vi "Little Digit Main.vi"() -> ()   [LabVIEW 2018]
uses:
  <vilib>/Instr/_visa.llb/VISA Configure Serial Port (Instr).vi
  <vilib>/Utility/inputDevices.llb/joystickAcquire.vi
  <vilib>/Utility/inputDevices.llb/closeJoystick.vi
  <vilib>/ptbypt/NI_PtbyPt.lvlib
panel:
  out "Elbow Degrees":dbl format="%.2f"
  out "Shoulder Degrees":dbl format="%.2f"
  in  "Vector Mode":bool=TRUE
  out "Shoulder Power":dbl
  out "Y axis":i32
  out "Z axis":i32
  out "Elbow power":dbl
  out "joystick info":T1(array[cluster])=[{"axes total"=6, "buttons total"=2, "pov total"=0, "device name"="SpaceNavigator"}, {"axes total"=8, "buttons total"=128, "pov total"=0, "device name"="Tetherscript Virtual Controller"}, {"axes total"=7, "buttons total"=4, "pov total"=1, "device name"="3Dconnexion KMJ Emulator"}]
  in  "OK Button":bool
  out "Lap Times":dbl[](array[numeric])
  out "Elapsed Time (s)":dbl=6.446096897125244
  out "Rotation Counts":i32=123
  out "Shoulder Counts":i32=65
  out "Elbow Counts":i32=112
  out "Wrist Counts":i32=80
  out "axis info":T2={"X axis"=-2, "Y axis"=-2, "Z axis"=-2, "X axis rotation"=-2, "Y axis rotation"=-2, "Z axis rotation"=-2, "U axis"=-2, "V axis"=-2}
  in  "stop":bool
  # "Little Digit\nTeam 5013"
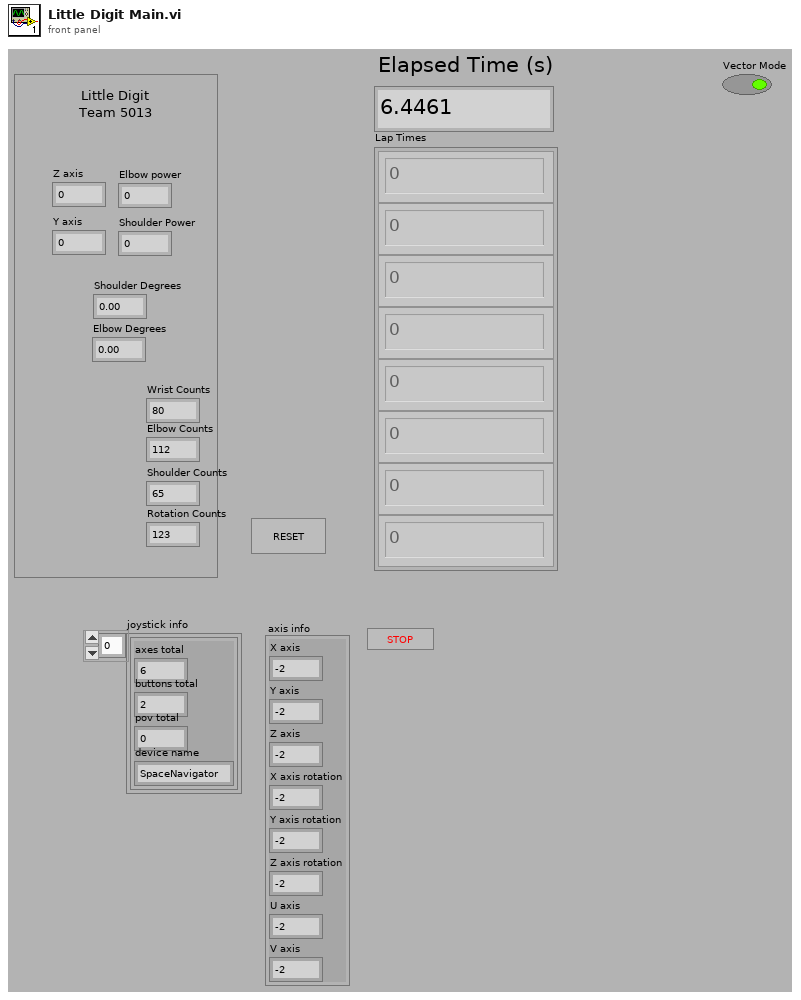
[diagram p1: front panel]
types:
  T1 = cluster{"axes total":u32, "buttons total":u32, "pov total":u32, "device name":string}[]
  T2 = cluster{"X axis":i32, "Y axis":i32, "Z axis":i32, "X axis rotation":i32, "Y axis rotation":i32, "Z axis rotation":i32, "U axis":i32, "V axis":i32}
  T3 = cluster{"button 1":bool, "button 2":bool, "button 3":bool, "button 4":bool, "button 5":bool, "button 6":bool, "button 7":bool, "button 8":bool, "button 9":bool, "button 10":bool, "button 11":bool, "button 12":bool, "button 13":bool, "button 14":bool, "button 15":bool, "button 16":bool, "button 17":bool, "button 18":bool, "button 19":bool, "button 20":bool, "button 21":bool, "button 22":bool, "button 23":bool, "button 24":bool, "button 25":bool, "button 26":bool, "button 27":bool, "button 28":bool, "button 29":bool, "button 30":bool, "button 31":bool, "button 32":bool}
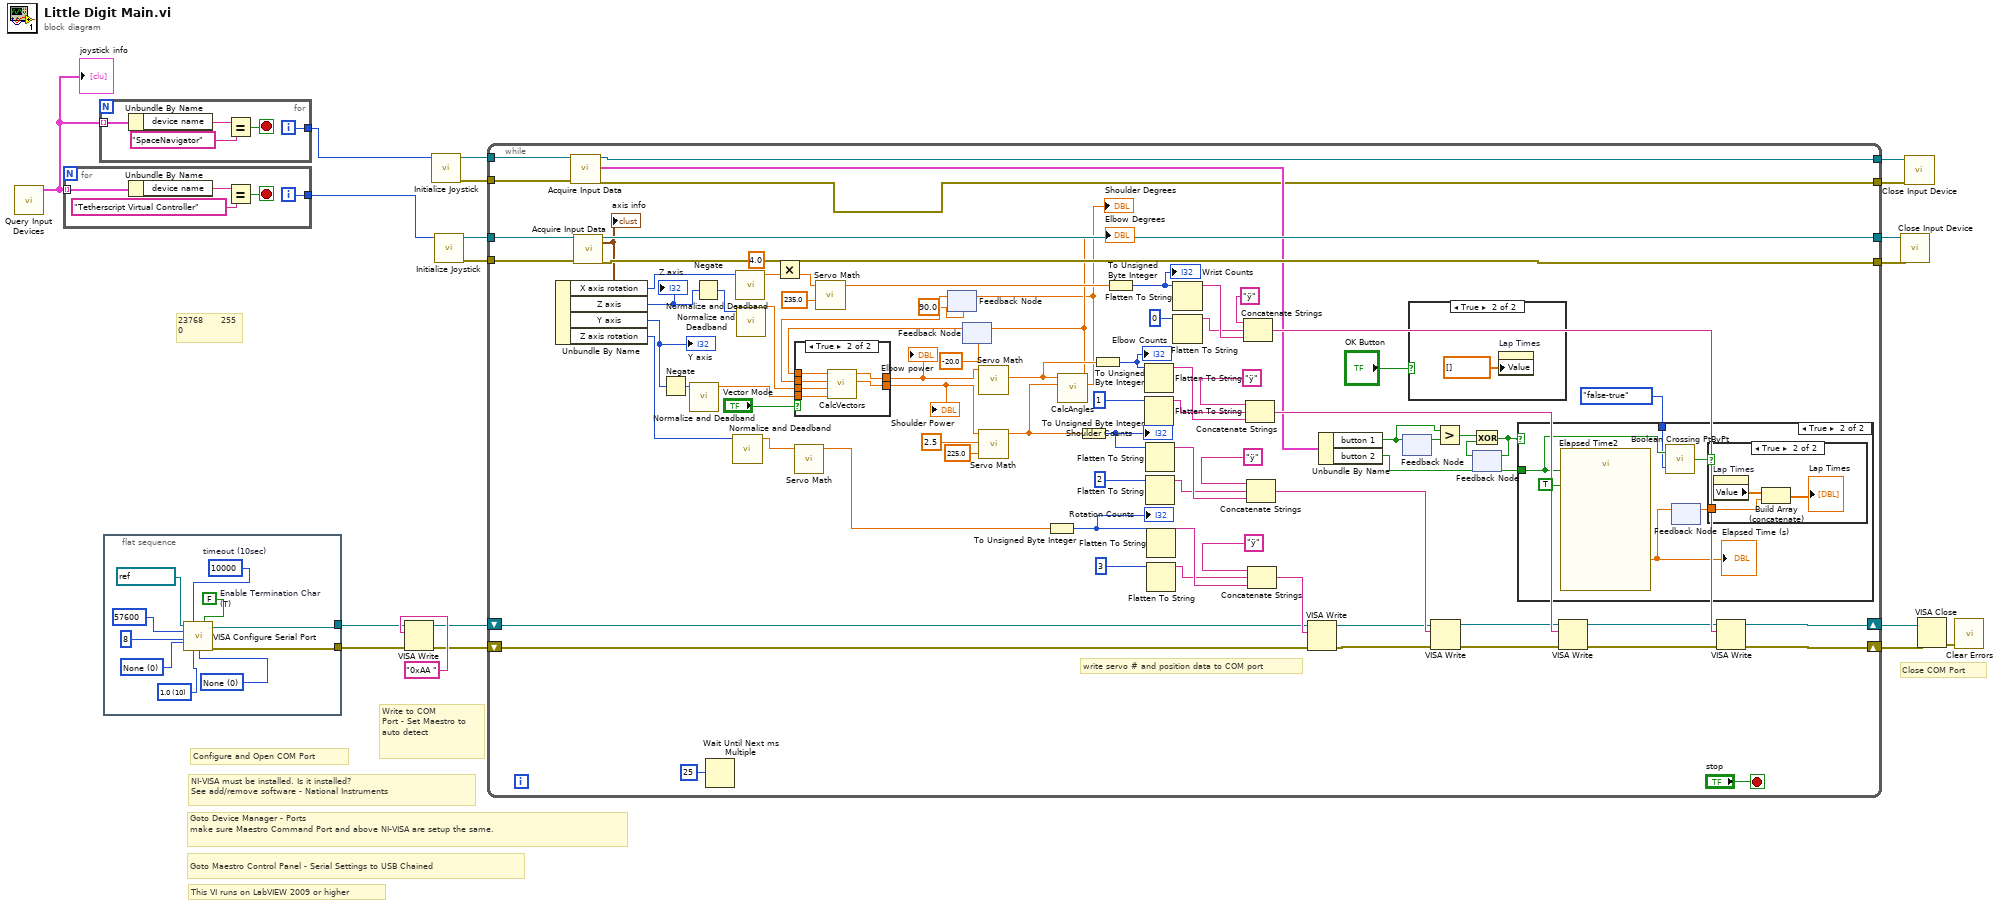
[diagram p0: block diagram]
diagram:
  # "23768      255\n0"
  # "This VI runs on LabVIEW 2009 or higher"
  # "Goto Maestro Control Panel - Serial Settings to USB Chained"
  # "Close COM Port"
  # "Configure and Open COM Port"
  # "Goto Device Manager - Ports \nmake sure Maestro Command Port and above NI-VISA are setup the same."
  # "NI-VISA must be installed. Is it installed?\nSee add/remove software - National Instruments"
  # "Write to COM \nPort - Set Maestro to auto detect"
  n1 = call <vilib>:"Query Input Devices.vi"() -> ("joystick info"=w3:T1)  [unwired: 8 in, 3 out]
  "joystick info" <- w3
  n2 = for {
    tunnel: w3 -> [w24] mode=indexing
    tunnel: [w20] -> w2
    i -> [w20]
    stop <- w21 stop-if-true
    n3 = Unbundle By Name(w24) -> ("device name"=w23:string)
    n4 = Equal?(x=w23, y="Tetherscript Virtual Controller") -> (x = y?=w21:bool)
  }
  n5 = for {
    tunnel: w3 -> [w29] mode=indexing
    tunnel: [w25] -> w1
    i -> [w25]
    stop <- w26 stop-if-true
    n6 = Unbundle By Name(w29) -> ("device name"=w28:string)
    n7 = Equal?(x=w28, y="SpaceNavigator") -> (x = y?=w26:bool)
  }
  n8 = flat-sequence {
    tunnel: [w31] -> w7
    tunnel: [w30] -> w9
    frame #0 {
      w32 = u16 0 items=["None"=0, "XON/XOFF"=1, "RTS/CTS"=2, "DTR/DSR"=4] ("flow control")
      w33 = u16 10 items=["1.0"=10, "1.5"=15, "2.0"=20] ("stop bits")
      w34 = u16 0 items=["None", "Odd", "Even", "Mark", "Space"] ("parity")
      w37 = FALSE  # Enable Termination Char (T)
      w38 = u32 10000  # timeout (10sec)
      n9 = call-poly "VISA Configure Serial Port"("VISA resource name"=refnum<visa-resource-name> "COM6", "timeout (10sec)"=w38, "Enable Termination\nChar (T)"=w37, "baud rate (9600)"=u32 57600 ("baud rate"), "data bits (8)"=u16 8 ("data bits"), "parity (0:none)"=w34, "stop bits (10: 1 bit)"=w33, "flow control (0:none)"=w32) -> ("VISA resource name out"=w31:refnum<visa-resource-name>, "error out"=w30:errorcluster)  [unwired: 1 in, 5 out]
    }
  }
  n10 = VISA Write(VISA resource name=w7, write buffer="0xAA ", error in (no error)=w9) -> (VISA resource name out=w6:refnum<visa-resource-name>, error out=w5:errorcluster)  [unwired: 1 out]
  n11 = call <vilib>:"Initialize Joystick.vi"("device index"=w1) -> ("error out"=w15:errorcluster, "device ID"=w14:refnum<k1>)  [unwired: 9 in]
  n12 = call <vilib>:"Initialize Joystick.vi"("device index"=w2) -> ("error out"=w18:errorcluster, "device ID"=w19:refnum<k1>)  [unwired: 9 in]
  n13 = while {
    tunnel: w19 -> [w117]
    tunnel: w18 -> [w116]
    tunnel: [w115] -> w17
    tunnel: [w114] -> w16
    tunnel: w14 -> [w77]
    tunnel: w15 -> [w78]
    tunnel: [w75] -> w13
    tunnel: [w74] -> w12
    shift-right: [w51] -> w10
    shift-left: w6 -> [w50]
    shift-right: [w52] -> w11
    shift-left: w5 -> [w49]
    stop <- "stop" stop-if-true
    # "write servo # and position data to COM port"
    n14 = call-poly <vilib>:"Acquire Input Data.vi"("device ID"=w77, "error in (no error)"=w78) -> ("device ID"=w75:refnum<k1>, "button info"=w76:T3, "error out"=w74:errorcluster)  [unwired: 13 in, 2 out]
    n15 = call-poly <vilib>:"Acquire Input Data.vi"("device ID"=w117, "error in (no error)"=w116) -> ("device ID"=w115:refnum<k1>, "axis info"=w113:T2, "error out"=w114:errorcluster)  [unwired: 13 in, 2 out]
    "axis info" <- w113
    n16 = Unbundle By Name(w113) -> ("X axis rotation"=w61:i32, "Z axis"=w92:i32, "Y axis"=w91:i32, "Z axis rotation"=w57:i32)
    "Z axis" <- w92
    "Y axis" <- w91
    n17 = Negate(x=w91) -> (-x=w55:i32)
    n18 = call "Normalize and Deadband.vi"("Numeric in"=w55) -> ("Numeric out"=w48:dbl)  [unwired: 10 in]
    n19 = Negate(x=w92) -> (-x=w58:i32)
    n20 = Wait Until Next ms Multiple(millisecond multiple=25) -> ()  [unwired: 1 out]
    n21 = call "Normalize and Deadband.vi"("Numeric in"=w57) -> ("Numeric out"=w56:dbl)  [unwired: 10 in]
    n22 = call "Normalize and Deadband.vi"("Numeric in"=w61) -> ("Numeric out"=w60:dbl)  [unwired: 10 in]
    n23 = call "Normalize and Deadband.vi"("Numeric in"=w58) -> ("Numeric out"=w59:dbl)  [unwired: 10 in]
    n24 = Multiply(x=4.0, y=w60) -> (x*y=w54:dbl)
    n25 = call "Servo Math.vi"("X axis rotation"=w56) -> ("Numeric"=w90:dbl)  [unwired: 10 in]
    n26 = call "Servo Math.vi"("upper limit"=235.0, "X axis rotation"=w54) -> ("Numeric"=w93:dbl)  [unwired: 9 in]
    n27 = feedback #1(90.0 ("Shoulder Degrees")) -> (w64:dbl)
    n28 = feedback #2(-20.0 ("Elbow Degrees")) -> (w66:dbl)
    n29 = case shown="True" "Vector Mode" {
      tunnel: [w123 w129] -> w69
      tunnel: [w122 w128] -> w68
      tunnel: w66 -> [_ w127]
      tunnel: w64 -> [_ w126]
      tunnel: w59 -> [w123 w125]
      tunnel: w48 -> [w122 w124]
      frame False {
      }
      frame True {
        n30 = call "CalcVectors.vi"("In/out"=w124, "Up/down"=w125, "Shoulder Degrees"=w126, "Elbow Degrees"=w127) -> ("Shoulder Power"=w128:dbl, "Elbow power"=w129:dbl)  [unwired: 6 in]
      }
    }
    "Elbow power" <- w69
    "Shoulder Power" <- w68
    n31 = call "Servo Math.vi"("X axis rotation"=w69) -> ("Numeric"=w71:dbl)  [unwired: 10 in]
    n32 = call "Servo Math.vi"("upper limit"=225.0, "Multipy Factor"=2.5, "X axis rotation"=w68) -> ("Numeric"=w70:dbl)  [unwired: 8 in]
    n33 = To Unsigned Byte Integer(number=w90) -> (unsigned 8bit integer=w45:u8)
    "Rotation Counts" <- w45
    n34 = call "CalcAngles.vi"("Shoulder Y"=w70, "Elbow X"=w71) -> ("Shoulder Degrees"=w65:dbl, "Elbow Degrees"=w67:dbl)  [unwired: 8 in]
    "Shoulder Degrees" <- w65
    "Elbow Degrees" <- w67
    n35 = feedback-in #1(w65) -> ()
    n36 = feedback-in #2(w67) -> ()
    n37 = To Unsigned Byte Integer(number=w70) -> (unsigned 8bit integer=w46:u8)
    "Shoulder Counts" <- w46
    n38 = To Unsigned Byte Integer(number=w71) -> (unsigned 8bit integer=w44:u8)
    "Elbow Counts" <- w44
    n39 = To Unsigned Byte Integer(number=w93) -> (unsigned 8bit integer=w43:u8)
    "Wrist Counts" <- w43
    n40 = Flatten To String(anything=w44) -> (data string=w99:string)  [unwired: 1 in, 4 out]
    n41 = Flatten To String(anything=u8 1 ("position")) -> (data string=w98:string)  [unwired: 1 in, 4 out]
    n42 = Flatten To String(anything=w46) -> (data string=w97:string)  [unwired: 1 in, 4 out]
    n43 = Flatten To String(anything=u8 2 ("position")) -> (data string=w96:string)  [unwired: 1 in, 4 out]
    n44 = Flatten To String(anything=w45) -> (data string=w95:string)  [unwired: 1 in, 4 out]
    n45 = Flatten To String(anything=u8 3 ("position")) -> (data string=w94:string)  [unwired: 1 in, 4 out]
    n46 = Flatten To String(anything=w43) -> (data string=w101:string)  [unwired: 1 in, 4 out]
    n47 = Flatten To String(anything=u8 0 ("position")) -> (data string=w100:string)  [unwired: 1 in, 4 out]
    n48 = Concatenate Strings("ÿ", w100, w101) -> (w103:string)
    n49 = Concatenate Strings("ÿ", w98, w99) -> (w104:string)
    n50 = Concatenate Strings("ÿ", w96, w97) -> (w105:string)
    n51 = Concatenate Strings("ÿ", w94, w95) -> (w106:string)
    n52 = VISA Write(VISA resource name=w50, write buffer=w106, error in (no error)=w49) -> (VISA resource name out=w89:refnum<visa-resource-name>, error out=w87:errorcluster)  [unwired: 1 out]
    n53 = Unbundle By Name(w76) -> ("button 1"=w82:bool, "button 2"=w84:bool)
    n54 = feedback-in #3(w82) -> ()
    n55 = feedback #3() -> (w83:bool)  [unwired: 1 in]
    n56 = case shown="True" "OK Button" {
      frame False {
      }
      frame True {
        n57 = property on="Lap Times" class="Arr (strict)"("Value"=dbl[] [] ("Lap Times")) -> ()  [unwired: 2 in, 2 out]
      }
    }
    n58 = VISA Write(VISA resource name=w89, write buffer=w105, error in (no error)=w87) -> (VISA resource name out=w88:refnum<visa-resource-name>, error out=w86:errorcluster)  [unwired: 1 out]
    n59 = Greater?(x=w82, y=w83) -> (0:w81:bool)
    n60 = feedback #4() -> (w80:bool)  [unwired: 1 in]
    n61 = Exclusive Or(1:w80, 2:w81) -> (0:w79:bool)
    n62 = feedback-in #4(w79) -> ()
    n63 = case shown="True" w79 {
      tunnel: w84 -> [_ w135]
      tunnel: enum16{"either", "false-true", "true-false"}."false-true" ("direction") -> [_ w133]
      frame False {
      }
      frame True {
        n64 = call "Elapsed Time2"("Reset"=w135, "Auto Reset"=TRUE) -> ("Elapsed Time (s)"=w132:dbl)  [unwired: 10 in, 7 out]
        "Elapsed Time (s)" <- w132
        n65 = call <vilib>:"Boolean Crossing PtByPt.vi"("direction"=w133, "input"=w135) -> ("crossing"=w134:bool)  [unwired: 1 in]
        n66 = feedback #5() -> (w131:dbl)  [unwired: 1 in]
        n67 = feedback-in #5(w132) -> ()
        n68 = case shown="True" w134 {
          tunnel: w131 -> [_ w138]
          frame False {
          }
          frame True {
            n69 = property on="Lap Times" class="Arr (strict)"() -> ("Value"=w139:dbl[])  [unwired: 2 in, 2 out]
            n70 = Build Array (concatenate)(w139, w138) -> (→"Lap Times":dbl[])
          }
        }
      }
    }
    n71 = VISA Write(VISA resource name=w88, write buffer=w104, error in (no error)=w86) -> (VISA resource name out=w102:refnum<visa-resource-name>, error out=w85:errorcluster)  [unwired: 1 out]
    n72 = VISA Write(VISA resource name=w102, write buffer=w103, error in (no error)=w85) -> (VISA resource name out=w51:refnum<visa-resource-name>, error out=w52:errorcluster)  [unwired: 1 out]
  }
  n73 = call-poly <vilib>:"Close Input Device.vi"("error in (no error)"=w16, "device ID"=w17) -> ()  [unwired: 8 in, 1 out]
  n74 = call-poly <vilib>:"Close Input Device.vi"("error in (no error)"=w12, "device ID"=w13) -> ()  [unwired: 8 in, 1 out]
  n75 = VISA Close(VISA resource name=w10, error in (no error)=w11) -> (error out=w4:errorcluster)
  n76 = call <vilib>:"Clear Errors.vi"("error in (no error)"=w4) -> ()  [unwired: 5 in, 2 out]
